vi "Init Pot.vi"(8 "error in (no error)":errorcluster, 11 "MCP4018 Digipot in":refnum<class "MCP4018 Digipot.lvclass">) -> (0 "error out":errorcluster, 2 "Data":string, 3 "MCP4018 Digipot out":refnum<class "MCP4018 Digipot.lvclass">)   [LabVIEW 2020, in "CTI-Peripheral.lvlib" / "MCP4018 Digipot.lvclass"]
uses:
  MCP4018 Digipot.lvclass
  MCP4018 Digipot.lvclass/MCP4018 Digipot.ctl
  CTI/I2C Connection/I2C Connection.lvclass/I2C Connection.ctl
  CTI/I2C Connection/I2C Connection.lvclass
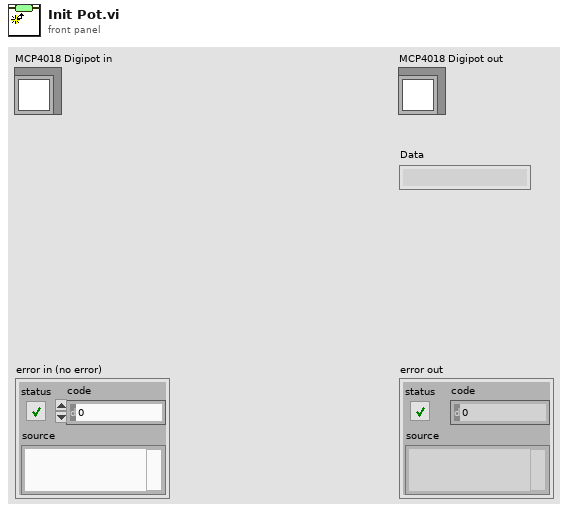
[diagram p1: front panel]
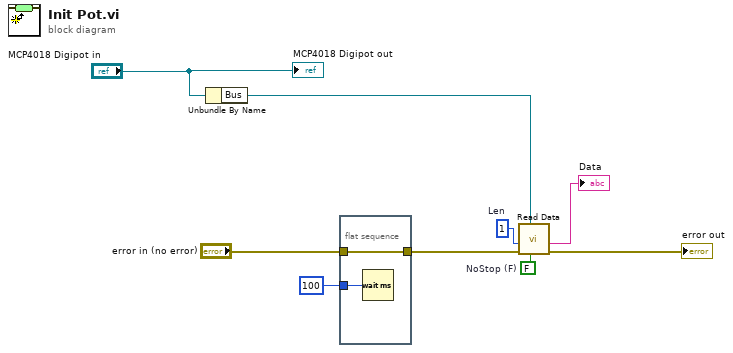
[diagram p0: block diagram]
diagram:
  w5 = FALSE  # NoStop (F)
  w6 = u8 1  # Len
  n1 = Unbundle By Name("MCP4018 Digipot in") -> ("Bus"=w2:refnum<class "I2C Connection.lvclass">)
  n2 = flat-sequence {
    tunnel: "error in (no error)" -> [w11]
    tunnel: [w11] -> w3
    tunnel: u32 100 ("milliseconds to wait") -> [w10]
    frame #0 {
      n3 = Wait (ms)(milliseconds to wait=w10) -> ()  [unwired: 1 out]
    }
  }
  n4 = call "Read Data.vi"("NoStop (F)"=w5, "I2C Connection"=w2, "error in (no error)"=w3, "Len"=w6) -> ("error out"=→"error out":errorcluster, "Data"=→"Data":string)  [unwired: 6 in]
  "MCP4018 Digipot out" <- "MCP4018 Digipot in"
